vi "CaLabGet_Main_Initialized.vi"(0 "CA Lab data":T2, 11 "Error in (no error)":errorcluster) -> (4 "PV Name (dup)":string[](array[string]), 6 "1rst Value (string)":string[](array[string]), 8 "1rst Value (number)":dbl[](array[numeric]), 10 "Value Array (number)":dbl[][](array[numeric]), 13 "Status":bool, 14 "PV Info":T1[](array[typedef]), 15 "Error out":errorcluster)   [LabVIEW 2018]
doc: "This is a VI for reading values of EPICS variables.\n\nINPUT:\n <b>CA Lab data</b>\n Cluster with preinitialized data\n <b>Error in (no error)</b>\n\nOUTPUT:\n <b>PV Name (dup)</b>\n name array of EPICS variables\n <b>1st Value(string)</b>\n value of variable as String\n shows first item of value array\n <b>1st Value(number)</b>\n value of variable as Double\n shows first item of value array\n <b>Value Array(number)</b>\n all values of variable in Double array\n <b>Error out</b>\n <b>PV Info</b>\n cluster array of full answer\n value array(number)\n PV name\n elements\n size of value array\n value array(string)\n all values of variable in string array\n value array(number)\n elements\n size of value array\n status(string)\n status of EPICS PV as String\n status(number)\n status of EPICS PV as Long\n severity(string)\n severity of EPICS PV as String\n severity(number)\n severity of EPICS PV as Long\n time stamp(string)\n stamp of EPICS PV time as String\n time stamp(number)\n stamp of EPICS PV as Long\n field names\n field values\n string array of requsted EPICS field values\n error IO\n <b>Status</b>\n FALSE: request successful\n TRUE: warnings or errors"
uses:
  <userlib>/caLab/PV Info.ctl
  <userlib>/caLab/lib/caLab.dll
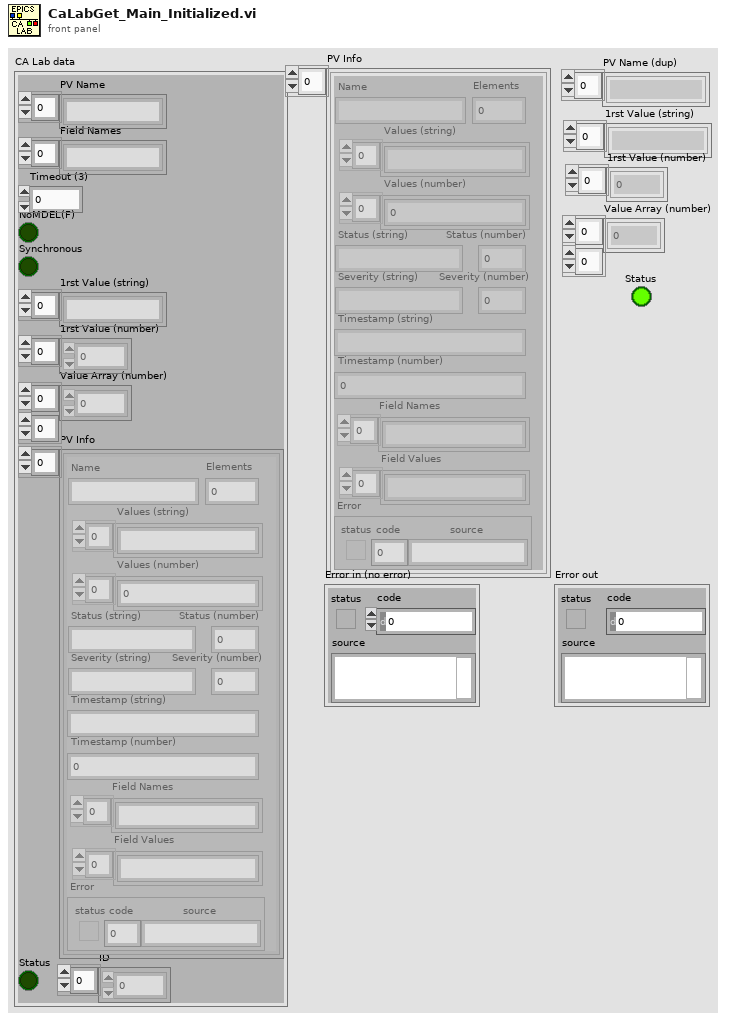
[diagram p1: front panel]
types:
  T1 = typedef "PV Info.ctl" = cluster{"Name":string, "Elements":i32, "Values (string)":string[], "Values (number)":dbl[], "Status (string)":string, "Status (number)":i16, "Severity (string)":string, "Severity (number)":i16, "Timestamp (string)":string, "Timestamp (number)":i32, "Field Names":string[], "Field Values":string[], "Error":errorcluster}
  T2 = cluster{"PV Name":string[], "Field Names":string[], "Timeout (3)":dbl, "NoMDEL(F)":bool, "Synchronous":bool, "1rst Value (string)":string[], "1rst Value (number)":dbl[], "Value Array (number)":dbl[][], "PV Info":T1[], "Status":bool, "ID":u64[]}
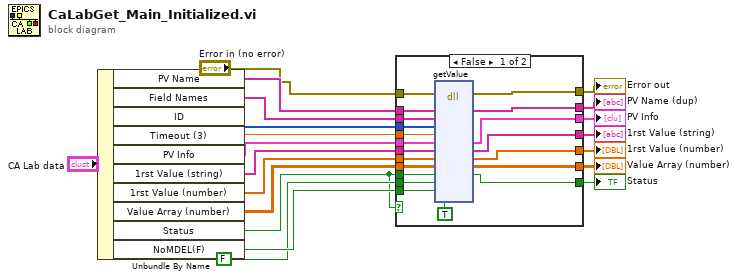
[diagram p0: block diagram]
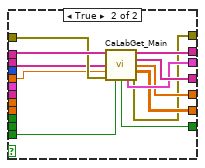
[diagram p2: hidden frame]
diagram:
  n1 = Unbundle By Name("CA Lab data") -> ("PV Name"=w20:string[], "Field Names"=w19:string[], "ID"=w18:u64[], "Timeout (3)"=w17:dbl, "PV Info"=w16:T1[], "1rst Value (string)"=w15:string[], "1rst Value (number)"=w14:dbl[], "Value Array (number)"=w13:dbl[][], "Status"=w1:bool, "NoMDEL(F)"=w12:bool)
  n2 = case shown="False" w1 {
    tunnel: w20 -> [w40 w52]
    tunnel: w19 -> [w39 w50]
    tunnel: w18 -> [w38 _]
    tunnel: w17 -> [w37 w49]
    tunnel: w16 -> [w36 _]
    tunnel: w15 -> [w35 _]
    tunnel: w14 -> [w34 _]
    tunnel: w13 -> [w33 _]
    tunnel: w1 -> [w32 _]
    tunnel: w12 -> [w31 w48]
    tunnel: FALSE ("FirstCall") -> [w30 _]
    tunnel: "Error in (no error)" -> [w29 w51]
    tunnel: [w27 w41] -> w8
    tunnel: [w26 w47] -> w7
    tunnel: [w25 w45] -> w6
    tunnel: [w24 w46] -> w5
    tunnel: [w23 w44] -> w4
    tunnel: [w22 w43] -> w3
    tunnel: [w21 w42] -> w2
    frame False {
      n3 = dll-call lib="D:/Program Files (x86)/National Instruments/LabVIEW 2018/user.lib/caLab/lib/calab.dll" fn="getValue" label="caLabGet"(error in=w29, "PVNameArray"=w40, "FieldNameArray"=w39, "IndexArray"=w38, "Timeout"=w37, "ResultClusterArray"=w36, "FirstStringValue"=w35, "FirstDoubleValue"=w34, "DoubleValueArray"=w33, "Status"=w32, "FirstCall"=w30, "NoMDEL"=w31, "IsInitialized"=TRUE) -> (error out=w27:errorcluster, "PVNameArray"=w26:string[], "ResultClusterArray"=w25:T1[], "FirstStringValue"=w24:string[], "FirstDoubleValue"=w23:dbl[], "DoubleValueArray"=w22:dbl[][], "Status"=w21:bool)  [unwired: 8 in, 2 out]
    }
    frame True {
      n4 = call <userlib>:"CaLabGet_Main.vi"("PV Name"=w52, "Field Names"=w50, "Timeout (3)"=w49, "error in (no error)"=w51, "NoMDEL(F)"=w48) -> ("PV Name (dup)"=w47:string[], "1rst Value (string)"=w46:string[], "1rst Value (number)"=w44:dbl[], "Value Array (number)"=w43:dbl[][], "Status"=w42:bool, "PV Info"=w45:T1[], "error out"=w41:errorcluster)  [unwired: 4 in]
    }
  }
  "Error out" <- w8
  "PV Name (dup)" <- w7
  "1rst Value (string)" <- w5
  "1rst Value (number)" <- w4
  "Value Array (number)" <- w3
  "Status" <- w2
  "PV Info" <- w6
